vi "ToString.vi"(8 "error in (no error)":errorcluster caption="错误输入（无错误）", 11 "Size 输入":refnum<class "Size.lvclass"> caption="DNL_LabVIEW Object in") -> (0 "error out":errorcluster caption="错误输出", 2 "ToString":string, 3 "Size 输出":refnum<class "Size.lvclass"> caption="DNL_LabVIEW Object out")   [LabVIEW 2011, in "Size.lvclass"]
uses:
  Size.lvclass
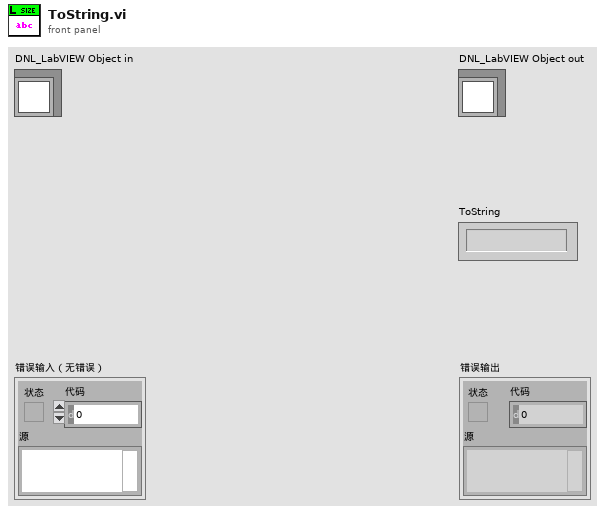
[diagram p1: front panel]
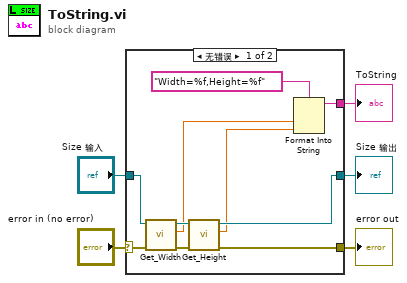
[diagram p0: block diagram]
diagram:
  n1 = case shown="无错误" "error in (no error)" {
    selector: "error in (no error)" -> [w12 w17]
    tunnel: [w10 w17] -> w4
    tunnel: [w13 w16] -> w2
    tunnel: "Size 输入" -> [w15 w16]
    tunnel: [w6 _] -> w1
    frame No Error {
      n2 = call "Get_Width.vi"("error in (no error)"=w12, "Size输入"=w15) -> ("error out"=w11:errorcluster, "Width"=w8:dbl, "Size输出"=w14:refnum<class "Size.lvclass">)  [unwired: 7 in]
      n3 = call "Get_Height.vi"("error in (no error)"=w11, "Size输入"=w14) -> ("error out"=w10:errorcluster, "Height"=w7:dbl, "Size输出"=w13:refnum<class "Size.lvclass">)  [unwired: 7 in]
      n4 = Format Into String(format string="Width=%f,Height=%f" ("格式字符串"), w8, w7) -> (resulting string=w6:string)  [unwired: 2 in, 1 out]
    }
    frame Error {
    }
  }
  "error out" <- w4
  "Size 输出" <- w2
  "ToString" <- w1
